vi "LDF Get Signal Value Str.vi"(7 "pValueStr":string, 9 "pSignalName":string, 10 "pFrameName":string, 11 "LDFHandle":u64) -> (1 "pSignalName out":string, 2 "pFrameName out":string, 3 "function return":i32, 5 "pValueStr out":string)   [LabVIEW 2010, in "ldf_parser.lvlib"]
doc: "int WINAPI LDF_GetSignalValueStr(long long LDFHandle, char* pFrameName, char* pSignalName, char* pValueStr);"
uses:
  ldf_parser.lvlib
  USB2XXX/trunk/USB2XXX/USB2XXX/vs2019/Release/USB2XXX.dll
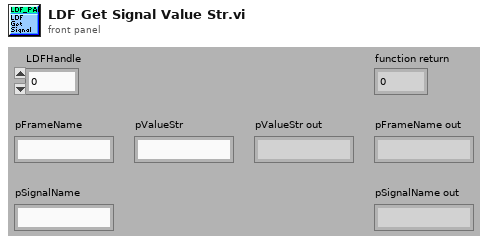
[diagram p1: front panel]
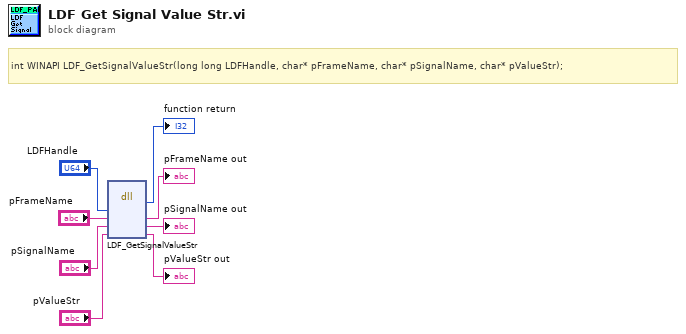
[diagram p0: block diagram]
diagram:
  # "int WINAPI LDF_GetSignalValueStr(long long LDFHandle, char* pFrameName, char* pSignalName, char* pValueStr);"
  n1 = dll-call lib="E:/Projects/USB2XXX/trunk/USB2XXX/USB2XXX/vs2019/Release/USB2XXX.*" fn="LDF_GetSignalValueStr"("LDFHandle"="LDFHandle", "pFrameName"="pFrameName", "pSignalName"="pSignalName", "pValueStr"="pValueStr") -> (→"function return":i32, "pFrameName"=→"pFrameName out":string, "pSignalName"=→"pSignalName out":string, "pValueStr"=→"pValueStr out":string)  [unwired: 4 in, 2 out]
